vi "Interval Timer.vi"() -> ()   [LabVIEW 2011]
panel:
  in  "Width (sec)":dbl(knob)=0.500001840510888 scale=0.0..1.0
  in  "Delay (sec)":dbl(knob)=0.20637723542731085 scale=0.0..1.0
  in  "Interval (sec)":dbl=2.0
  out "Waveform Chart":cluster{i16, i16}(graph)
  out "test":bool
  out "Relative Time":dbl
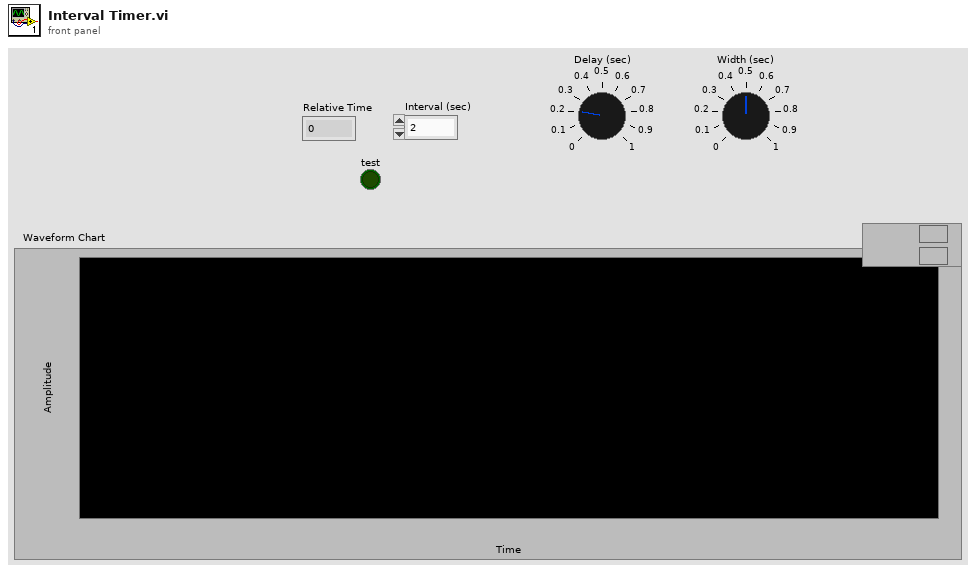
[diagram p1: front panel]
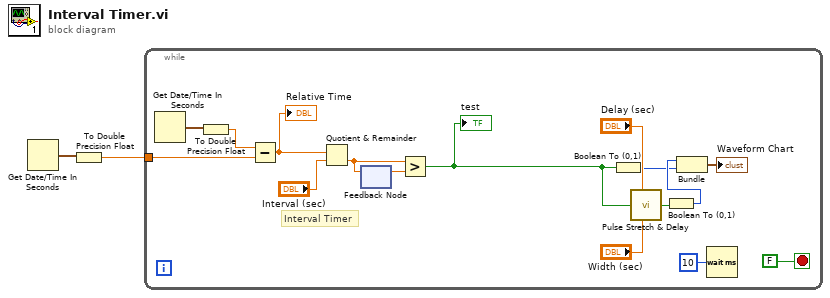
[diagram p0: block diagram]
diagram:
  n1 = Get Date/Time In Seconds() -> (seconds since 1Jan1904=w2:timestamp)
  n2 = To Double Precision Float(number=w2) -> (double precision float=w1:dbl)
  n3 = while {
    tunnel: w1 -> [w16]
    stop <- FALSE stop-if-true
    # "Interval Timer"
    n4 = Get Date/Time In Seconds() -> (seconds since 1Jan1904=w18:timestamp)
    n5 = To Double Precision Float(number=w18) -> (double precision float=w17:dbl)
    n6 = Subtract(x=w17, y=w16) -> (x-y=w13:dbl)
    "Relative Time" <- w13
    n7 = Quotient & Remainder(x=w13, y="Interval (sec)") -> (floor(x/y)=w12:dbl)  [unwired: 1 out]
    n8 = feedback-in #1(w12) -> ()
    n9 = feedback #1() -> (w11:dbl)  [unwired: 1 in]
    n10 = Greater?(x=w12, y=w11) -> (0:w3:bool)
    "test" <- w3
    n11 = Boolean To (0,1)(Boolean=w3) -> (0, 1=w4:i16)
    n12 = call "Pulse Stretch & Delay.vi"("Delay (sec)"="Delay (sec)", "In"=w3, "Width (sec)"="Width (sec)") -> ("Out"=w9:bool)  [unwired: 2 in]
    n13 = Boolean To (0,1)(Boolean=w9) -> (0, 1=w5:i16)
    n14 = Bundle(w5, w4) -> (→"Waveform Chart":cluster{i16, i16})  [unwired: 1 in]
    n15 = Wait (ms)(milliseconds to wait=u32 10) -> ()  [unwired: 1 out]
  }
